vi "Obtain Tag Bus Queue.vi"(8 "error in":errorcluster, 11 "data allocations":T1) -> (0 "error out":errorcluster, 2 "tag bus queues":T4, 3 "data allocations out":T1)   [LabVIEW 2013, in "J1939.lvlib"]
uses:
  J1939.lvlib
  API Types/Tag Bus Queues.ctl
  <vilib>/NI/Tag Bus/table/data table.ctl
  <vilib>/NI/Tag Bus Module Framework/channel/data tables.ctl
  <vilib>/NI/Tag Bus/dictionary/data dictionary.lvclass
  <vilib>/NI/Tag Bus/dictionary table pair.ctl
  <vilib>/NI/Tag Bus/table/data table.lvlib
  <vilib>/NI/Tag Bus/tag bus.lvlib
  <vilib>/NI/Tag Bus Module Framework/channel/TBM channel.lvclass
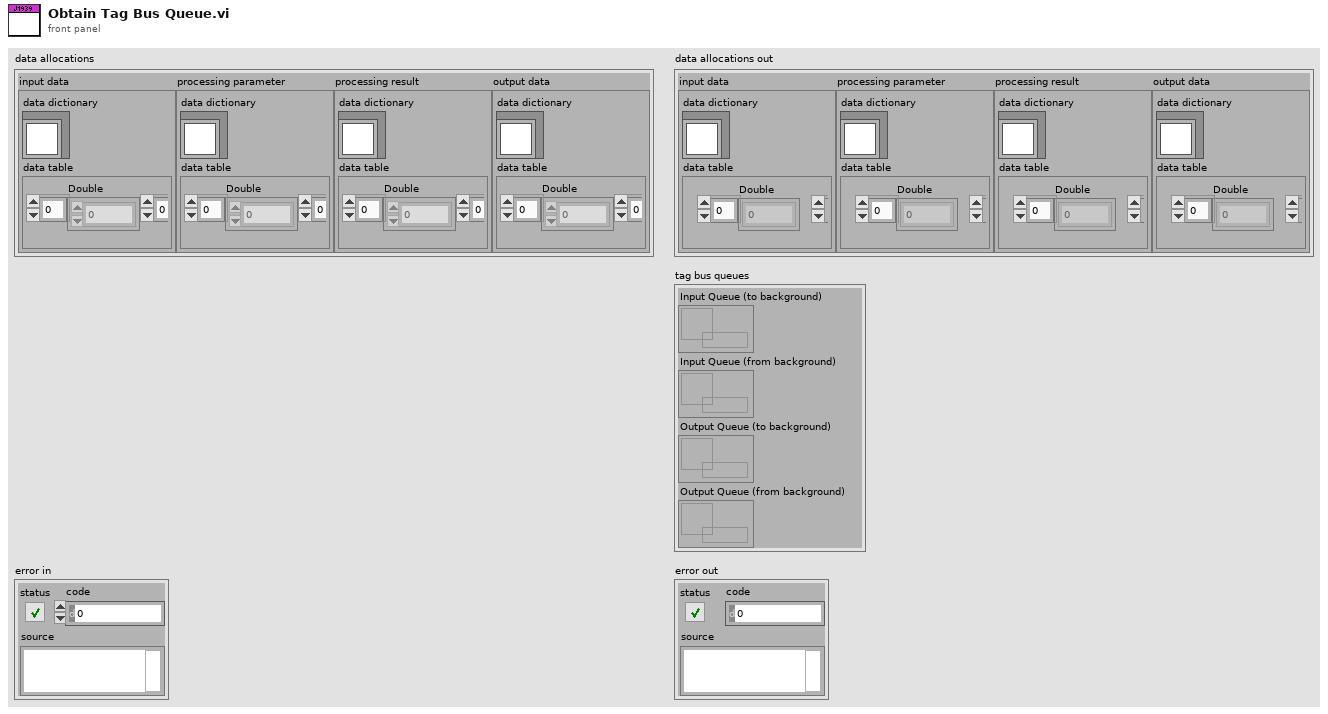
[diagram p1: front panel]
types:
  T1 = typedef "TBM channel.lvclass/data tables.ctl" = cluster{"input data":T2, "processing parameter":T2, "processing result":T2, "output data":T2}
  T2 = typedef "tag bus.lvlib/dictionary table pair.ctl" = cluster{"data dictionary":refnum<class "data dictionary.lvclass">, "data table":T3}
  T3 = typedef "tag bus.lvlib/data table.lvlib/data table.ctl" = cluster{"Double":dbl[], "Single":sgl[], "I64":i64[], "I32":i32[], "I16":i16[], "I8":i8[], "U64":u64[], "U32":u32[], "U16":u16[], "U8":u8[], "Boolean":bool[], "String":string[], "Array of Double":cluster{"DBL Array":dbl[]}[], "Array of Single":cluster{"SGL Array":sgl[]}[], "Array of I64":cluster{"I64 Array":i64[]}[], "Array of I32":cluster{"I32 Array":i32[]}[], "Array of I16":cluster{"I16 Array":i16[]}[], "Array of I8":cluster{"I8 Array":i8[]}[], "Array of U64":cluster{"U64 Array":u64[]}[], "Array of U32":cluster{"U32 Array":u32[]}[], "Array of U16":cluster{"U16 Array":u16[]}[], "Array of U8":cluster{"U8 Array":u8[]}[], "Array of Boolean":cluster{"Boolean Array":bool[]}[], "Array of String":cluster{"String Array":string[]}[]}
  T4 = typedef "J1939.lvlib/Tag Bus Queues.ctl" = cluster{"Input Queue (to background)":refnum<queue>, "Input Queue (from background)":refnum<queue>, "Output Queue (to background)":refnum<queue>, "Output Queue (from background)":refnum<queue>}
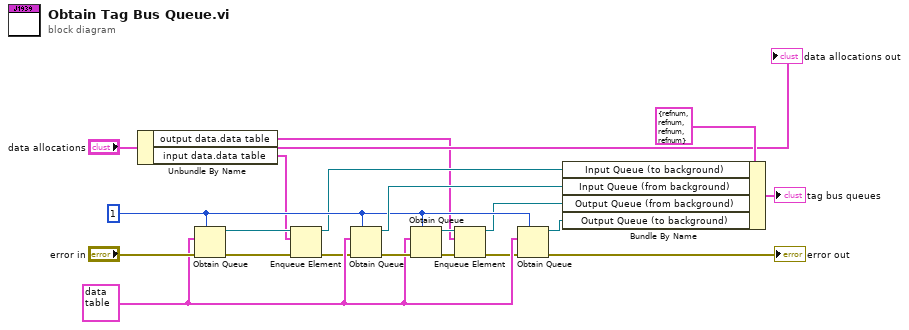
[diagram p0: block diagram]
diagram:
  w10 = 1 ("max queue size (-1, unlimited)")
  w11 = T3 {"Double"=[], "Single"=[], "I64"=[], "I32"=[], "I16"=[], "I8"=[], "U64"=[], "U32"=[], "U16"=[], "U8"=[], "Boolean"=[], "String"=[], "Array of Double"=[], "Array of Single"=[], "Array of I64"=[], "Array of I32"=[], "Array of I16"=[], "Array of I8"=[], "Array of U64"=[], "Array of U32"=[], "Array of U16"=[], "Array of U8"=[], "Array of Boolean"=[], "Array of String"=[]} ("data table")
  n1 = Unbundle By Name("data allocations") -> ("output data.data table"=w2:T3, "input data.data table"=w1:T3)
  n2 = Obtain Queue(max queue size (-1, unlimited)=w10, element data type=w11, error in (no error)="error in") -> (queue out=w8:refnum<queue>, error out=w15:errorcluster)  [unwired: 2 in, 1 out]
  n3 = Enqueue Element(queue=w8, element=w1, error in (no error)=w15) -> (queue out=w7:refnum<queue>, error out=w9:errorcluster)  [unwired: 1 in, 1 out]
  n4 = Obtain Queue(max queue size (-1, unlimited)=w10, element data type=w11, error in (no error)=w9) -> (queue out=w12:refnum<queue>, error out=w17:errorcluster)  [unwired: 2 in, 1 out]
  n5 = Obtain Queue(max queue size (-1, unlimited)=w10, element data type=w11, error in (no error)=w17) -> (queue out=w5:refnum<queue>, error out=w16:errorcluster)  [unwired: 2 in, 1 out]
  n6 = Enqueue Element(queue=w5, element=w2, error in (no error)=w16) -> (queue out=w4:refnum<queue>, error out=w6:errorcluster)  [unwired: 1 in, 1 out]
  n7 = Obtain Queue(max queue size (-1, unlimited)=w10, element data type=w11, error in (no error)=w6) -> (queue out=w13:refnum<queue>, error out=→"error out":errorcluster)  [unwired: 2 in, 1 out]
  n8 = Bundle By Name(cluster=T4 {"Input Queue (to background)"=refnum, "Input Queue (from background)"=refnum, "Output Queue (to background)"=refnum, "Output Queue (from background)"=refnum} ("tag bus queues 2"), "Input Queue (to background)"=w7, "Input Queue (from background)"=w12, "Output Queue (from background)"=w4, "Output Queue (to background)"=w13) -> (→"tag bus queues":T4)
  "data allocations out" <- "data allocations"
